vi "NH485_Test.vi"() -> ()   [LabVIEW 2014]
uses:
  NH485_Test_Globals.vi
panel:
  in  "Address":u32[](array[numeric])=[0]
  out "HumArray":dbl[](array[numeric]) format="%.2f"
  out "TempArray":dbl[](array[numeric]) format="%.2f"
  in  "Comport(s)":refnum<visa-resource-name>[](array[refnum])=["ASRL2::INSTR"]
  in  "stop":bool
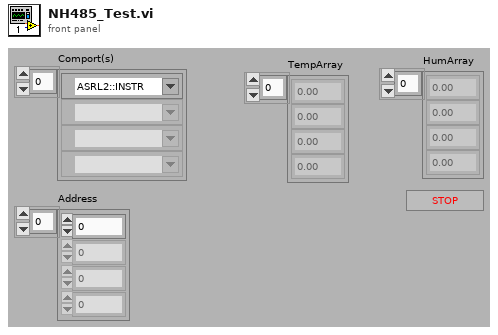
[diagram p1: front panel]
types:
  T1 = typedef "NH485 Object Reference.ctl" = refnum<k1>
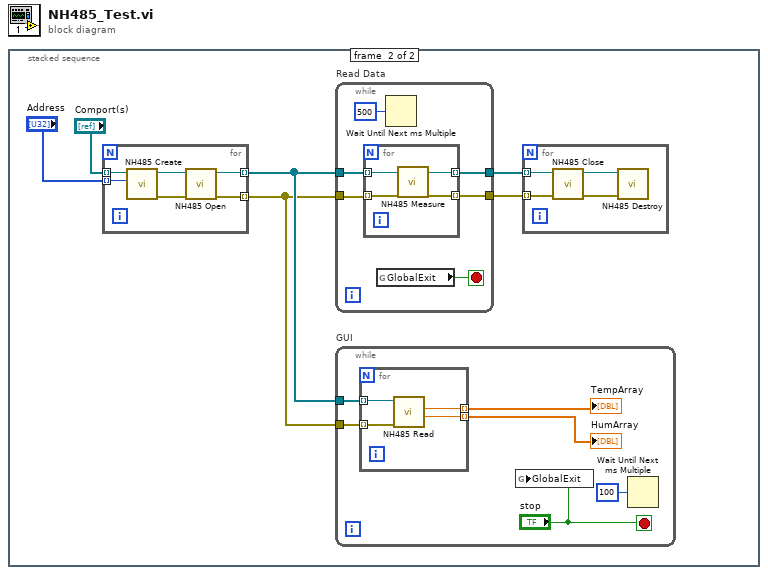
[diagram p0: block diagram]
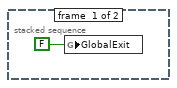
[diagram p2: hidden frame]
diagram:
  n1 = stacked-sequence {
    frame #0 {
      n2 = global write "NH485_Test_Globals.vi" "GlobalExit"(FALSE ("GlobalExit")) -> ()
    }
    frame #1 {
      n3 = for {
        tunnel: "Comport(s)" -> [w27] mode=indexing
        tunnel: [w24] -> w4 mode=indexing
        tunnel: [w23] -> w3 mode=indexing
        tunnel: "Address" -> [w22] mode=indexing
        n4 = call "NH485 Create.vi"("Address"=w22, "VISA Resource Name"=w27) -> ("error out"=w25:errorcluster, "reference"=w26:T1)  [unwired: 4 in]
        n5 = call "NH485 Open.vi"("error in (no error)"=w25, "reference"=w26) -> ("error out"=w23:errorcluster, "duplicate reference"=w24:T1)  [unwired: 8 in]
      }
      n6 = while "Read Data" {
        tunnel: w4 -> [w17]
        tunnel: w3 -> [w16]
        tunnel: [w14] -> w6
        tunnel: [w13] -> w5
        stop <- w12 stop-if-true
        n7 = for {
          tunnel: [w21] -> w13 mode=indexing
          tunnel: [w20] -> w14 mode=indexing
          tunnel: w17 -> [w19] mode=indexing
          tunnel: w16 -> [w18] mode=indexing
          n8 = call "NH485 Measure.vi"("error in (no error)"=w18, "reference"=w19) -> ("error out"=w21:errorcluster, "duplicate reference"=w20:T1)  [unwired: 8 in]
        }
        n9 = global read "NH485_Test_Globals.vi" "GlobalExit"() -> (w12:bool)
        n10 = Wait Until Next ms Multiple(millisecond multiple=u32 500) -> ()  [unwired: 1 out]
      }
      n11 = while "GUI" {
        tunnel: w3 -> [w32]
        tunnel: w4 -> [w31]
        stop <- "stop" stop-if-true
        n12 = for {
          tunnel: w32 -> [w37] mode=indexing
          tunnel: w31 -> [w36] mode=indexing
          tunnel: [w35] -> w30 mode=indexing
          tunnel: [w34] -> w29 mode=indexing
          n13 = call "NH485 Read.vi"("error in (no error)"=w37, "reference"=w36) -> ("Humidity"=w34:dbl, "Temp"=w35:dbl)  [unwired: 6 in, 2 out]
        }
        "TempArray" <- w30
        "HumArray" <- w29
        n14 = global write "NH485_Test_Globals.vi" "GlobalExit"("stop") -> ()
        n15 = Wait Until Next ms Multiple(millisecond multiple=u32 100) -> ()  [unwired: 1 out]
      }
      n16 = for {
        tunnel: w6 -> [w11] mode=indexing
        tunnel: w5 -> [w10] mode=indexing
        n17 = call "NH485 Close.vi"("error in (no error)"=w10, "reference"=w11) -> ("error out"=w9:errorcluster, "duplicate reference"=w8:T1)  [unwired: 8 in]
        n18 = call "NH485 Destroy.vi"("error in (no error)"=w9, "reference"=w8) -> ()  [unwired: 5 in, 1 out]
      }
    }
  }
